vi "MAIN.vi"() -> ()   [LabVIEW 2020]
uses:
  GlobIndSw1.vi
panel:
  in  "Median Filter Rank":i32=25
  out "Oscilloscope Capture":waveform(dbl)[](graph)
  out "start time":timestamp
  out "Started":bool
  out "Elapsed time (minutes)":dbl
  out "error out":errorcluster
  in  "error in (no error)":errorcluster
  out "TEST#   |  Elapsed Time (minutes)":dbl[][](array[numeric])
  out "Inductive Switching :\nTotal Test Time (minutes)":dbl
  out "Cluster : Tf":cluster{"Tf (ns)":dbl, "DONE Tf":bool} {"Tf (ns)" format="%_12f"}
  out "Cluster : Tdoff":cluster{"Tdoff (ns)":dbl, "DONE Tdoff":bool} {"Tdoff (ns)" format="%_12f"}
  out "Cluster : Eoff":cluster{"Eoff (uj)":dbl, "DONE Eoff":bool} {"Eoff (uj)" format="%_12f"}
  out "Cluster : Dv/Dt ON":T1 {"Dv/Dt ON (V/us)" format="%_12f"}
  out "Cluster : Eon":cluster{"Eon (uj)":dbl, "DONE Eon":bool} {"Eon (uj)" format="%_12f"}
  out "Cluster : Di/Dt ON":T2 {"Di/Dt ON (A/us)" format="%_12f"}
  out "Cluster : Dv/DT OFF":T3 {"Dv/DT OFF (V/us)" format="%_12f"}
  out "Cluster : Di/Dt OFF":T4 {"Di/Dt OFF (A/us)" format="%_12f"}
  out "Cluster : Tr":cluster{"Tr (ns)":dbl, "DONE Tr":bool} {"Tr (ns)" format="%_12f"}
  out "Cluster : Tdon":cluster{"Tdon (ns)":dbl, "DONE Tdon":bool} {"Tdon (ns)" format="%_12f"}
  in  "Finish?":bool
  in  "Cluster : Setting":T5={"VGE (V)"=0.0, "VCE (V)"=0.0, "ICE (A)"=0.0, "TEKTRONIX"="", "PROJECT #"="", "TEMPERATURE (C)"=0.0, "RG (Ohm)"=0.0, "DUT #"=1, "REQUEST #"="", "TEST #"=1}
  out "CURRENT RESULT Array":dbl[](array[numeric])
  out "ALL RESULT Array":dbl[][](array[numeric])
  in  "START TEST":bool
  # "PRODUCED BY : AFIQAH HASBULLAH ( SBN CZ ENG : 2021)"
  # "AC MODULE : Inductive Switching"
  # "Column 2"
  # "Column 3"
  # "Column 4"
  # "Column 5"
  # "Column 6"
  # "Column 7"
  # "Column 8"
  # "Column 9"
  # "Column 10"
  # "Column 11"
  # "Column 12"
  # "Column 13"
  # "Column 14"
  # "Column 15"
  # "Column 16"
  # "Column 18"
  # "Column 19"
  # "Column 20"
  # "Column 21"
  # "Column 22"
  # "Column 23"
  # "Column 24"
  # "Column 25"
  # "Column 0"
  # "Column 1"
  # "----------------Already Calculated---------------------"
  # "Tdon\n(ns)"
  # "Tr\n(ns)"
  # "Tdoff\n(ns)"
  # "Tf\n(ns)"
  # "Eon\n(uj)"
  # "Eoff\n(uj)"
  # "di/dt (on)\nA/us"
  # "di/dt (off)\nA/us"
  # "dv/dt (on)\nV/us"
  # "dv/dt (off)\nV/us"
  # "NULL\n(Separator)"
  # "on\ndi (A)"
  # "on\ndt (ns)"
  # "off\ndi (A)"
  # "off\ndt (ns)"
  # "on\ndv (V)"
  # "on\ndt (ns)"
  # "off\ndv (V)"
  # "off\ndt (ns)"
  # "Vce"
  # "Ice"
  # "Vge"
  # "Rg"
  # "Temperature"
  # "DUT  #"
  # "TEST #"
  # "< Press 2 times >"
  # "Column 2"
  # "Column 3"
  # "Column 4"
  # "Column 5"
  # "Column 6"
  # "Column 7"
  # "Column 8"
  # "Column 9"
  # "Column 10"
  # "Column 11"
  # "Column 12"
  # "Column 13"
  # "Column 14"
  # "Column 15"
  # "Column 16"
  # "Column 18"
  # "Column 19"
  # "Column 20"
  # "Column 21"
  # "Column 22"
  # "Column 23"
  # "Column 24"
  # "Column 25"
  # "Column 0"
  # "Column 1"
  # "----------------Already Calculated---------------------"
  # "Tdon\n(ns)"
  # "Tr\n(ns)"
  # "Tdoff\n(ns)"
  # "Tf\n(ns)"
  # "Eon\n(uj)"
  # "Eoff\n(uj)"
  # "di/dt (on)\nA/us"
  # "di/dt (off)\nA/us"
  # "dv/dt (on)\nV/us"
  # "dv/dt (off)\nV/us"
  # "NULL\n(Separator)"
  # "on\ndi (A)"
  # "on\ndt (ns)"
  # "off\ndi (A)"
  # "off\ndt (ns)"
  # "on\ndv (V)"
  # "on\ndt (ns)"
  # "off\ndv (V)"
  # "off\ndt (ns)"
  # "TEST #"
  # "Vce"
  # "Ice"
  # "Vge"
  # "Rg"
  # "Temperature"
  # "DUT  #"
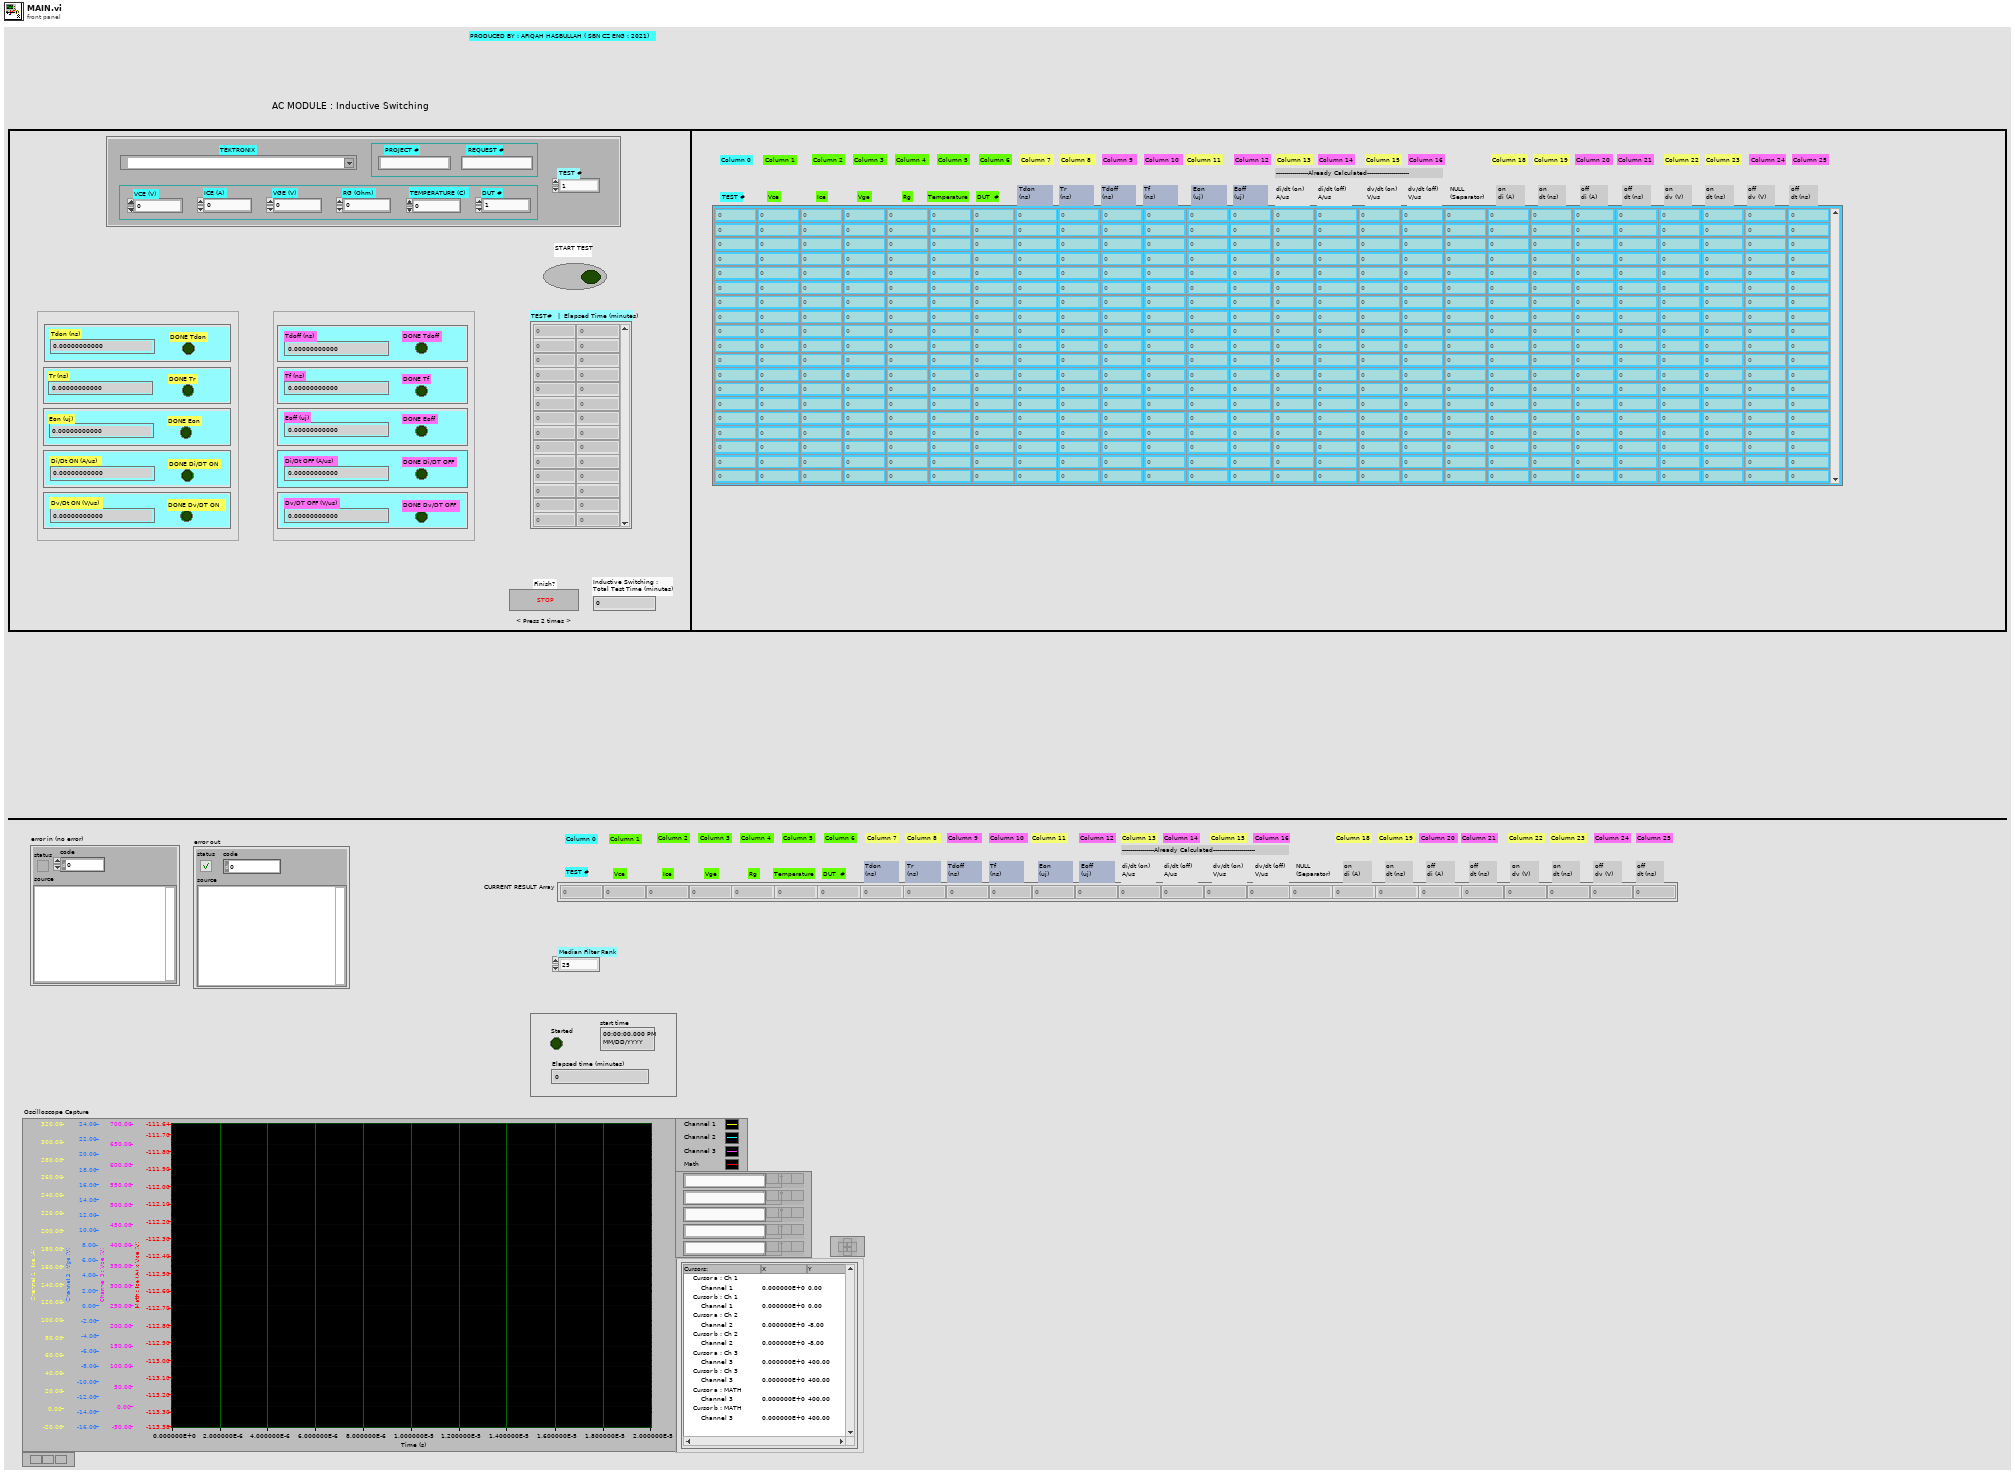
[diagram p1: front panel]
types:
  T1 = cluster{"Dv/Dt ON (V/us)":dbl, "DONE Dv/DT ON":bool}
  T2 = cluster{"Di/Dt ON (A/us)":dbl, "DONE Di/DT ON":bool}
  T3 = cluster{"Dv/DT OFF (V/us)":dbl, "DONE Dv/DT OFF":bool}
  T4 = cluster{"Di/Dt OFF (A/us)":dbl, "DONE Di/DT OFF":bool}
  T5 = cluster{"VGE (V)":dbl, "VCE (V)":dbl, "ICE (A)":dbl, "TEKTRONIX":refnum<visa-resource-name>, "PROJECT #":string, "TEMPERATURE (C)":dbl, "RG (Ohm)":dbl, "DUT #":i32, "REQUEST #":string, "TEST #":i32}
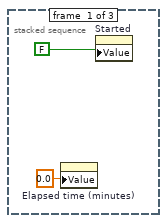
[diagram p2: hidden frame]
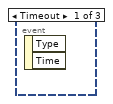
[diagram p4: hidden frame]
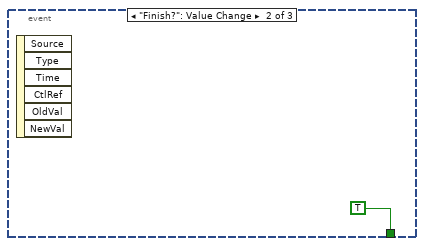
[diagram p5: hidden frame]
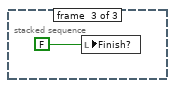
[diagram p7: hidden frame]
diagram:
  w23 = errorcluster {"status"=FALSE, "code"=0, "source"=""} ("error out")
  w4 = 0.0 ("Inductive Switching :\nTotal Test Time (minutes)")
  w5 = FALSE ("START TEST")
  w24 = cluster{"Tdon (ns)":dbl, "DONE Tdon":bool} {"Tdon (ns)"=0.0, "DONE Tdon"=FALSE} ("Cluster : Tdon")
  n1 = local read "Cluster : Setting"() -> (w19:T5)
  n2 = Bundle By Name(cluster=w19, "TEST #"=1, "DUT #"=1) -> (w20:T5)
  n3 = local write "Median Filter Rank"(25 ("Median Filter Rank")) -> ()
  n4 = local write "Cluster : Setting"(w20) -> ()
  n5 = flat-sequence {
    tunnel: [w26] -> w3
    tunnel: w3 -> [w27]
    tunnel: [w28] -> w22
    tunnel: w22 -> [w303]
    tunnel: [w301] -> w21
    tunnel: w21 -> [w328]
    frame #0 {
      # "IN"
      n6 = local read "error in (no error)"() -> (w26:errorcluster)
      n7 = Wait (ms)(milliseconds to wait=u32 100) -> ()  [unwired: 1 out]
    }
    frame #1 {
      # "Main Loop"
      n8 = while {
        shift-right: [w31] -> w28
        shift-left: w27 -> [w30]
        stop <- w33 stop-if-true
        n9 = local read "START TEST"() -> (w34:bool)
        n10 = case shown="True" w34 {
          tunnel: w30 -> [w35 w61]
          tunnel: [w35 w58] -> w31
          frame False {
          }
          frame True {
            # "Reset Start Button"
            # "Increment TEST# & DUT#"
            # "Update Data in All Result Array"
            # "OFF region Test"
            # "ON region Test"
            # "Header Information"
            # "Initialize"
            n11 = flat-sequence {
              tunnel: [w68] -> w62
              tunnel: w61 -> [w68]
              tunnel: [w93] -> w63
              tunnel: w62 -> [w93]
              tunnel: w63 -> [w148]
              tunnel: [w147] -> w57
              tunnel: [w126] -> w55
              tunnel: [w127] -> w54
              tunnel: [w128] -> w53
              tunnel: [w129] -> w52
              tunnel: [w136] -> w51
              tunnel: [w137] -> w50
              tunnel: [w135] -> w49
              tunnel: [w138] -> w48
              tunnel: [w139] -> w47
              tunnel: w57 -> [w199]
              tunnel: [w199] -> w56
              tunnel: w55 -> [w179]
              tunnel: w54 -> [w177]
              tunnel: w53 -> [w175]
              tunnel: w52 -> [w173]
              tunnel: w51 -> [w171]
              tunnel: w50 -> [w169]
              tunnel: w49 -> [w167]
              tunnel: w48 -> [w165]
              tunnel: w47 -> [w163]
              tunnel: w56 -> [w223]
              tunnel: [w222] -> w46
              tunnel: [w201] -> w44
              tunnel: [w202] -> w43
              tunnel: [w203] -> w42
              tunnel: [w204] -> w41
              tunnel: [w211] -> w40
              tunnel: [w212] -> w39
              tunnel: [w210] -> w38
              tunnel: [w213] -> w37
              tunnel: [w214] -> w36
              tunnel: w46 -> [w274]
              tunnel: [w274] -> w45
              tunnel: w44 -> [w254]
              tunnel: w43 -> [w252]
              tunnel: w42 -> [w250]
              tunnel: w41 -> [w248]
              tunnel: w40 -> [w246]
              tunnel: w39 -> [w244]
              tunnel: w38 -> [w242]
              tunnel: w37 -> [w240]
              tunnel: w36 -> [w238]
              tunnel: w45 -> [w277]
              tunnel: [w277] -> w59
              tunnel: [w283] -> w60
              tunnel: w59 -> [w283]
              tunnel: [w293] -> w58
              tunnel: w60 -> [w293]
              frame #0 {
                w69 = FALSE ("DONE Tdon")
                w70 = 0.0 ("Tdon (ns)")
                n12 = local read "Cluster : Di/Dt ON"() -> (w84:T2)
                n13 = local read "Cluster : Dv/Dt ON"() -> (w82:T1)
                n14 = local read "Cluster : Eon"() -> (w87:cluster{"Eon (uj)":dbl, "DONE Eon":bool})
                n15 = local read "Cluster : Tdon"() -> (w89:cluster{"Tdon (ns)":dbl, "DONE Tdon":bool})
                n16 = Bundle By Name(cluster=w84, "Di/Dt ON (A/us)"=w70, "DONE Di/DT ON"=w69) -> (w85:T2)
                n17 = local write "Oscilloscope Capture"(waveform(dbl)[] [] ("Oscilloscope Capture")) -> ()
                n18 = local read "Cluster : Tr"() -> (w90:cluster{"Tr (ns)":dbl, "DONE Tr":bool})
                n19 = Bundle By Name(cluster=w82, "Dv/Dt ON (V/us)"=w70, "DONE Dv/DT ON"=w69) -> (w83:T1)
                n20 = Bundle By Name(cluster=w87, "Eon (uj)"=w70, "DONE Eon"=w69) -> (w86:cluster{"Eon (uj)":dbl, "DONE Eon":bool})
                n21 = Bundle By Name(cluster=w89, "Tdon (ns)"=w70, "DONE Tdon"=w69) -> (w88:cluster{"Tdon (ns)":dbl, "DONE Tdon":bool})
                n22 = Bundle By Name(cluster=w90, "Tr (ns)"=w70, "DONE Tr"=w69) -> (w91:cluster{"Tr (ns)":dbl, "DONE Tr":bool})
                n23 = local write "Cluster : Di/Dt ON"(w85) -> ()
                n24 = local write "Cluster : Dv/Dt ON"(w83) -> ()
                n25 = local write "Cluster : Eon"(w86) -> ()
                n26 = local write "Cluster : Tdon"(w88) -> ()
                n27 = local write "Cluster : Tr"(w91) -> ()
                n28 = Initialize Array(0.0 ("element"), 26 ("dimension size")) -> (w65:dbl[])
                n29 = local write "CURRENT RESULT Array"(w65) -> ()
                n30 = local read "Cluster : Di/Dt OFF"() -> (w77:T4)
                n31 = local read "Cluster : Tdoff"() -> (w74:cluster{"Tdoff (ns)":dbl, "DONE Tdoff":bool})
                n32 = local read "Cluster : Eoff"() -> (w76:cluster{"Eoff (uj)":dbl, "DONE Eoff":bool})
                n33 = local read "Cluster : Tf"() -> (w71:cluster{"Tf (ns)":dbl, "DONE Tf":bool})
                n34 = local read "Cluster : Dv/DT OFF"() -> (w80:T3)
                n35 = Bundle By Name(cluster=w77, "Di/Dt OFF (A/us)"=w70, "DONE Di/DT OFF"=w69) -> (w78:T4)
                n36 = Bundle By Name(cluster=w74, "Tdoff (ns)"=w70, "DONE Tdoff"=w69) -> (w73:cluster{"Tdoff (ns)":dbl, "DONE Tdoff":bool})
                n37 = Bundle By Name(cluster=w76, "Eoff (uj)"=w70, "DONE Eoff"=w69) -> (w75:cluster{"Eoff (uj)":dbl, "DONE Eoff":bool})
                n38 = Bundle By Name(cluster=w71, "Tf (ns)"=w70, "DONE Tf"=w69) -> (w72:cluster{"Tf (ns)":dbl, "DONE Tf":bool})
                n39 = Bundle By Name(cluster=w80, "Dv/DT OFF (V/us)"=w70, "DONE Dv/DT OFF"=w69) -> (w79:T3)
                n40 = local write "Cluster : Tdoff"(w73) -> ()
                n41 = local write "Cluster : Di/Dt OFF"(w78) -> ()
                n42 = local write "Cluster : Eoff"(w75) -> ()
                n43 = local write "Cluster : Tf"(w72) -> ()
                n44 = local write "Cluster : Dv/DT OFF"(w79) -> ()
                n45 = Wait (ms)(milliseconds to wait=u32 400) -> ()  [unwired: 1 out]
              }
              frame #1 {
                # "Column 6 = DUT#"
                # "Column 5 = Temperature"
                # "Column 4 = RG"
                # "Column 3 = VGE"
                # "Column 2 = ICE"
                # "Column 1 = VCE"
                # "Column 0 = TEST#"
                n46 = local read "Cluster : Setting"() -> (w123:T5)
                n47 = Wait (ms)(milliseconds to wait=u32 400) -> ()  [unwired: 1 out]
                n48 = Unbundle By Name(w123) -> ("TEST #"=w119:i32, "ICE (A)"=w111:dbl, "VGE (V)"=w107:dbl, "VCE (V)"=w115:dbl, "RG (Ohm)"=w103:dbl, "TEMPERATURE (C)"=w99:dbl, "DUT #"=w95:i32)
                n49 = local read "CURRENT RESULT Array"() -> (w122:dbl[])
                n50 = local read "CURRENT RESULT Array"() -> (w116:dbl[])
                n51 = local read "CURRENT RESULT Array"() -> (w114:dbl[])
                n52 = local read "Median Filter Rank"() -> (w92:i32)
                n53 = local read "CURRENT RESULT Array"() -> (w108:dbl[])
                n54 = local read "CURRENT RESULT Array"() -> (w106:dbl[])
                n55 = local read "CURRENT RESULT Array"() -> (w100:dbl[])
                n56 = local read "CURRENT RESULT Array"() -> (w98:dbl[])
                n57 = Replace Array Subset(array=w122, new element=w119, index=0) -> (w121:dbl[])
                n58 = Replace Array Subset(array=w116, new element=w115, index=1) -> (w117:dbl[])
                n59 = Replace Array Subset(array=w114, new element=w111, index=2) -> (w113:dbl[])
                n60 = global write "GlobIndSw1.vi" "Median Filter Rank"(w92) -> ()
                n61 = Replace Array Subset(array=w108, new element=w107, index=3) -> (w109:dbl[])
                n62 = Replace Array Subset(array=w106, new element=w103, index=4) -> (w105:dbl[])
                n63 = Replace Array Subset(array=w100, new element=w99, index=5) -> (w101:dbl[])
                n64 = Replace Array Subset(array=w98, new element=w95, index=6) -> (w97:dbl[])
                n65 = local write "CURRENT RESULT Array"(w121) -> ()
                n66 = local write "CURRENT RESULT Array"(w117) -> ()
                n67 = local write "CURRENT RESULT Array"(w113) -> ()
                n68 = local write "CURRENT RESULT Array"(w109) -> ()
                n69 = local write "CURRENT RESULT Array"(w105) -> ()
                n70 = local write "CURRENT RESULT Array"(w101) -> ()
                n71 = local write "CURRENT RESULT Array"(w97) -> ()
              }
              frame #2 {
                n72 = local read "Cluster : Setting"() -> (w161:T5)
                n73 = Unbundle By Name(w161) -> ("TEKTRONIX"=w146:refnum<visa-resource-name>, "PROJECT #"=w145:string, "REQUEST #"=w144:string, "TEST #"=w150:i32, "ICE (A)"=w142:dbl, "VGE (V)"=w141:dbl, "VCE (V)"=w140:dbl)
                n74 = Format Value(format string="%d", value (0)=w150) -> (output string=w143:string)  [unwired: 1 in]
                n75 = call "f_ON_Region.vi"("VISA Resource Name"=w146, "Project #"=w145, "Request #"=w144, "TEST #"=w143, "ICE"=w142, "VGE"=w141, "VCE"=w140, "error in (no error)"=w148) -> ("Tdon (ns)"=w139:dbl, "Di (A)"=w129:dbl, "Tr (ns)"=w138:dbl, "Dt (ns)"=w128:dbl, "Di/Dt (A/us)"=w137:dbl, "Dv/Dt (V/us)"=w136:dbl, "Eon (uj)"=w135:dbl, "Dv (V)"=w127:dbl, "Dt (ns) 2"=w126:dbl, "DONE Tdon"=w134:bool, "DONE Tr"=w133:bool, "DONE Di/Dt ON"=w132:bool, "DONE Dv/Dt ON"=w131:bool, "DONE Eon"=w130:bool, "Oscilloscope Capture"=w124:waveform(dbl)[], "error out"=w147:errorcluster)  [unwired: 4 in]
                n76 = local write "Oscilloscope Capture"(w124) -> ()
                n77 = local read "Cluster : Dv/Dt ON"() -> (w160:T1)
                n78 = local read "Cluster : Di/Dt ON"() -> (w158:T2)
                n79 = Bundle By Name(cluster=w160, "Dv/Dt ON (V/us)"=w136, "DONE Dv/DT ON"=w131) -> (w159:T1)
                n80 = Bundle By Name(cluster=w158, "Di/Dt ON (A/us)"=w137, "DONE Di/DT ON"=w132) -> (w157:T2)
                n81 = local read "Cluster : Eon"() -> (w155:cluster{"Eon (uj)":dbl, "DONE Eon":bool})
                n82 = local read "Cluster : Tr"() -> (w152:cluster{"Tr (ns)":dbl, "DONE Tr":bool})
                n83 = local read "Cluster : Tdon"() -> (w153:cluster{"Tdon (ns)":dbl, "DONE Tdon":bool})
                n84 = Bundle By Name(cluster=w155, "Eon (uj)"=w135, "DONE Eon"=w130) -> (w156:cluster{"Eon (uj)":dbl, "DONE Eon":bool})
                n85 = Bundle By Name(cluster=w152, "Tr (ns)"=w138, "DONE Tr"=w133) -> (w151:cluster{"Tr (ns)":dbl, "DONE Tr":bool})
                n86 = Bundle By Name(cluster=w153, "Tdon (ns)"=w139, "DONE Tdon"=w134) -> (w154:cluster{"Tdon (ns)":dbl, "DONE Tdon":bool})
                n87 = local write "Cluster : Dv/Dt ON"(w159) -> ()
                n88 = local write "Cluster : Di/Dt ON"(w157) -> ()
                n89 = local write "Cluster : Eon"(w156) -> ()
                n90 = local write "Cluster : Tr"(w151) -> ()
                n91 = local write "Cluster : Tdon"(w154) -> ()
                n92 = Wait (ms)(milliseconds to wait=u32 300) -> ()  [unwired: 1 out]
              }
              frame #3 {
                # "Column 23 = Dt2"
                # "Column 22 = Dv"
                # "Column 19 = Dt"
                # "Column 18 = Di"
                # "Column 15 = DvDtON"
                # "Column 13 = DiDtON"
                # "Column 11 = Eon"
                # "Column 8 = Tr"
                # "Column 7 = Tdon"
                n93 = Wait (ms)(milliseconds to wait=u32 2000) -> ()  [unwired: 1 out]
                n94 = local read "CURRENT RESULT Array"() -> (w181:dbl[])
                n95 = local read "CURRENT RESULT Array"() -> (w184:dbl[])
                n96 = local read "CURRENT RESULT Array"() -> (w188:dbl[])
                n97 = local read "CURRENT RESULT Array"() -> (w185:dbl[])
                n98 = local read "CURRENT RESULT Array"() -> (w189:dbl[])
                n99 = local read "CURRENT RESULT Array"() -> (w197:dbl[])
                n100 = local read "CURRENT RESULT Array"() -> (w193:dbl[])
                n101 = local read "CURRENT RESULT Array"() -> (w196:dbl[])
                n102 = local read "CURRENT RESULT Array"() -> (w192:dbl[])
                n103 = Replace Array Subset(array=w181, new element=w163, index=7) -> (w182:dbl[])
                n104 = Replace Array Subset(array=w184, new element=w165, index=8) -> (w183:dbl[])
                n105 = Replace Array Subset(array=w188, new element=w169, index=13) -> (w187:dbl[])
                n106 = Replace Array Subset(array=w185, new element=w167, index=11) -> (w186:dbl[])
                n107 = Replace Array Subset(array=w189, new element=w171, index=15) -> (w190:dbl[])
                n108 = Replace Array Subset(array=w197, new element=w173, index=18) -> (w198:dbl[])
                n109 = Replace Array Subset(array=w193, new element=w177, index=22) -> (w194:dbl[])
                n110 = Replace Array Subset(array=w196, new element=w175, index=19) -> (w195:dbl[])
                n111 = Replace Array Subset(array=w192, new element=w179, index=23) -> (w191:dbl[])
                n112 = local write "CURRENT RESULT Array"(w182) -> ()
                n113 = local write "CURRENT RESULT Array"(w183) -> ()
                n114 = local write "CURRENT RESULT Array"(w187) -> ()
                n115 = local write "CURRENT RESULT Array"(w186) -> ()
                n116 = local write "CURRENT RESULT Array"(w190) -> ()
                n117 = local write "CURRENT RESULT Array"(w198) -> ()
                n118 = local write "CURRENT RESULT Array"(w194) -> ()
                n119 = local write "CURRENT RESULT Array"(w195) -> ()
                n120 = local write "CURRENT RESULT Array"(w191) -> ()
              }
              frame #4 {
                n121 = local read "Cluster : Setting"() -> (w225:T5)
                n122 = Unbundle By Name(w225) -> ("TEKTRONIX"=w221:refnum<visa-resource-name>, "PROJECT #"=w220:string, "REQUEST #"=w219:string, "TEST #"=w236:i32, "ICE (A)"=w217:dbl, "VGE (V)"=w216:dbl, "VCE (V)"=w215:dbl)
                n123 = Format Value(format string="%d", value (0)=w236) -> (output string=w218:string)  [unwired: 1 in]
                n124 = call "f_OFF_Region.vi"("VISA Resource Name"=w221, "Project #"=w220, "Request #"=w219, "TEST #"=w218, "ICE"=w217, "VGE"=w216, "VCE"=w215, "error in (no error)"=w223) -> ("Tdoff (ns)"=w214:dbl, "Di (A)"=w204:dbl, "Tf (ns)"=w213:dbl, "Dt (ns)"=w203:dbl, "Di/Dt (A/us)"=w212:dbl, "Dv/Dt (V/us)"=w211:dbl, "Eoff (uj)"=w210:dbl, "Dv (V)"=w202:dbl, "Dt (ns) 2"=w201:dbl, "DONE Tdoff"=w209:bool, "DONE Tf"=w208:bool, "DONE Di/Dt OFF"=w207:bool, "DONE Dv/Dt OFF"=w206:bool, "DONE Eoff"=w205:bool, "error out"=w222:errorcluster)  [unwired: 5 in]
                n125 = local read "Cluster : Dv/DT OFF"() -> (w226:T3)
                n126 = local read "Cluster : Di/Dt OFF"() -> (w228:T4)
                n127 = Bundle By Name(cluster=w226, "Dv/DT OFF (V/us)"=w211, "DONE Dv/DT OFF"=w206) -> (w227:T3)
                n128 = Bundle By Name(cluster=w228, "Di/Dt OFF (A/us)"=w212, "DONE Di/DT OFF"=w207) -> (w229:T4)
                n129 = local read "Cluster : Eoff"() -> (w231:cluster{"Eoff (uj)":dbl, "DONE Eoff":bool})
                n130 = local read "Cluster : Tf"() -> (w234:cluster{"Tf (ns)":dbl, "DONE Tf":bool})
                n131 = local read "Cluster : Tdoff"() -> (w233:cluster{"Tdoff (ns)":dbl, "DONE Tdoff":bool})
                n132 = Bundle By Name(cluster=w231, "Eoff (uj)"=w210, "DONE Eoff"=w205) -> (w230:cluster{"Eoff (uj)":dbl, "DONE Eoff":bool})
                n133 = Bundle By Name(cluster=w234, "Tf (ns)"=w213, "DONE Tf"=w208) -> (w235:cluster{"Tf (ns)":dbl, "DONE Tf":bool})
                n134 = Bundle By Name(cluster=w233, "Tdoff (ns)"=w214, "DONE Tdoff"=w209) -> (w232:cluster{"Tdoff (ns)":dbl, "DONE Tdoff":bool})
                n135 = local write "Cluster : Dv/DT OFF"(w227) -> ()
                n136 = local write "Cluster : Di/Dt OFF"(w229) -> ()
                n137 = local write "Cluster : Eoff"(w230) -> ()
                n138 = local write "Cluster : Tf"(w235) -> ()
                n139 = local write "Cluster : Tdoff"(w232) -> ()
                n140 = Wait (ms)(milliseconds to wait=u32 300) -> ()  [unwired: 1 out]
              }
              frame #5 {
                # "Column 25 = Dt2"
                # "Column 24 = Dv"
                # "Column 21 = Dt"
                # "Column 20 = Di"
                # "Column 16 = DvDtOFF"
                # "Column 14 = DiDtOFF"
                # "Column 12 = Eoff"
                # "Column 10 = Tf"
                # "Column 9 = Tdoff"
                n141 = Wait (ms)(milliseconds to wait=u32 2000) -> ()  [unwired: 1 out]
                n142 = local read "CURRENT RESULT Array"() -> (w273:dbl[])
                n143 = local read "CURRENT RESULT Array"() -> (w270:dbl[])
                n144 = local read "CURRENT RESULT Array"() -> (w266:dbl[])
                n145 = local read "CURRENT RESULT Array"() -> (w269:dbl[])
                n146 = local read "CURRENT RESULT Array"() -> (w265:dbl[])
                n147 = local read "CURRENT RESULT Array"() -> (w257:dbl[])
                n148 = local read "CURRENT RESULT Array"() -> (w261:dbl[])
                n149 = local read "CURRENT RESULT Array"() -> (w258:dbl[])
                n150 = local read "CURRENT RESULT Array"() -> (w262:dbl[])
                n151 = Replace Array Subset(array=w273, new element=w238, index=9) -> (w272:dbl[])
                n152 = Replace Array Subset(array=w270, new element=w240, index=10) -> (w271:dbl[])
                n153 = Replace Array Subset(array=w266, new element=w244, index=14) -> (w267:dbl[])
                n154 = Replace Array Subset(array=w269, new element=w242, index=12) -> (w268:dbl[])
                n155 = Replace Array Subset(array=w265, new element=w246, index=16) -> (w264:dbl[])
                n156 = Replace Array Subset(array=w257, new element=w248, index=20) -> (w256:dbl[])
                n157 = Replace Array Subset(array=w261, new element=w252, index=24) -> (w260:dbl[])
                n158 = Replace Array Subset(array=w258, new element=w250, index=21) -> (w259:dbl[])
                n159 = Replace Array Subset(array=w262, new element=w254, index=25) -> (w263:dbl[])
                n160 = local write "CURRENT RESULT Array"(w272) -> ()
                n161 = local write "CURRENT RESULT Array"(w271) -> ()
                n162 = local write "CURRENT RESULT Array"(w267) -> ()
                n163 = local write "CURRENT RESULT Array"(w268) -> ()
                n164 = local write "CURRENT RESULT Array"(w264) -> ()
                n165 = local write "CURRENT RESULT Array"(w256) -> ()
                n166 = local write "CURRENT RESULT Array"(w260) -> ()
                n167 = local write "CURRENT RESULT Array"(w259) -> ()
                n168 = local write "CURRENT RESULT Array"(w263) -> ()
              }
              frame #6 {
                n169 = local read "Cluster : Setting"() -> (w282:T5)
                n170 = Unbundle By Name(w282) -> ("TEST #"=w276:i32)
                n171 = local read "CURRENT RESULT Array"() -> (w281:dbl[])
                n172 = local read "ALL RESULT Array"() -> (w280:dbl[][])
                n173 = Decrement(x=w276) -> (x-1=w275:i32)
                n174 = Replace Array Subset(array=w280, new element=w281, index (row)=w275) -> (w279:dbl[][])  [unwired: 1 in]
                n175 = local write "ALL RESULT Array"(w279) -> ()
                n176 = Wait (ms)(milliseconds to wait=u32 300) -> ()  [unwired: 1 out]
              }
              frame #7 {
                n177 = local read "Cluster : Setting"() -> (w291:T5)
                n178 = Unbundle By Name(w291) -> ("TEST #"=w290:i32, "DUT #"=w289:i32)
                n179 = Increment(x=w290) -> (x+1=w285:i32)
                n180 = Increment(x=w289) -> (x+1=w284:i32)
                n181 = local read "Cluster : Setting"() -> (w287:T5)
                n182 = Bundle By Name(cluster=w287, "TEST #"=w285, "DUT #"=w284) -> (w286:T5)
                n183 = local write "Cluster : Setting"(w286) -> ()
                n184 = Wait (ms)(milliseconds to wait=u32 200) -> ()  [unwired: 1 out]
              }
              frame #8 {
                n185 = local write "START TEST"(FALSE ("START TEST")) -> ()
                n186 = local write "Started"(FALSE ("START TEST")) -> ()
                n187 = Wait (ms)(milliseconds to wait=u32 1000) -> ()  [unwired: 1 out]
              }
            }
          }
        }
        n188 = Wait (ms)(milliseconds to wait=u32 100) -> ()  [unwired: 1 out]
        n189 = local read "Finish?"() -> (w33:bool)
      }
      n190 = Wait (ms)(milliseconds to wait=u32 100) -> ()  [unwired: 1 out]
    }
    frame #2 {
      # "Minutes"
      # "Export to Excel"
      n191 = local read "TEST#   |  Elapsed Time (minutes)"() -> (w308:dbl[][])
      n192 = local read "Cluster : Setting"() -> (w315:T5)
      n193 = Unbundle By Name(w315) -> ("TEST #"=w297:i32)
      n194 = Index Array(array=w308, index (col)=1 ("disabled index (col)")) -> (element=w306:dbl[])  [unwired: 1 in]
      n195 = Decrement(x=w297) -> (x-1=w296:i32)
      n196 = local read "ALL RESULT Array"() -> (w310:dbl[][])
      n197 = local read "Cluster : Setting"() -> (w319:T5)
      n198 = Split 1D Array(array=w306, index=w296) -> (first subarray=w305:dbl[])  [unwired: 1 out]
      n199 = Decrement(x=w297) -> (x-1=w311:i32)
      n200 = for {
        tunnel: w305 -> [w323] mode=indexing
        shift-right: [w322] -> w304
        shift-left: 0.0 -> [w321]
        shift-right: [w320] -> w300
        shift-left: w303 -> [w320]
        n201 = Add(x=w323, y=w321) -> (x+y=w322:dbl)
        n202 = local write "Inductive Switching :\nTotal Test Time (minutes)"(w322) -> ()
      }
      n203 = Unbundle By Name(w319) -> ("PROJECT #"=w318:string, "REQUEST #"=w317:string)
      n204 = Array Subset(array=w310, index (row)=0 ("index"), length (row)=w311, index (col)=0 ("index"), length (col)=26 ("length")) -> (w309:dbl[][])
      n205 = call "O_Data_to_Excel.vi"("error in (no error)"=w303, "ALL RESULT Array"=w309, "REQUEST #"=w317, "PROJECT #"=w318) -> ("error out"=w299:errorcluster)  [unwired: 7 in]
      n206 = Wait (ms)(milliseconds to wait=u32 100) -> ()  [unwired: 1 out]
      n207 = local write "Inductive Switching :\nTotal Test Time (minutes)"(w304) -> ()
      n208 = Merge Errors(w299, w300) -> (w298:errorcluster)
      n209 = while {
        shift-right: [w324] -> w301
        shift-left: w298 -> [w325]
        stop <- w326 stop-if-true
        n210 = call "Display Message to User"("error in (no error)"=w325) -> ("error out"=w324:errorcluster, "OK"=w326:bool)  [unwired: 9 in]
        n211 = Wait (ms)(milliseconds to wait=u32 100) -> ()  [unwired: 1 out]
      }
    }
    frame #3 {
      # "OUT"
      n212 = local write "error out"(w328) -> ()
      n213 = Wait (ms)(milliseconds to wait=u32 100) -> ()  [unwired: 1 out]
    }
  }
  n214 = Initialize Array(0.0 ("element"), 26 ("dimension size")) -> (→"CURRENT RESULT Array":dbl[])
  n215 = Initialize Array(0.0 ("element"), 100 ("dimension size"), 2 ("dimension size")) -> (→"TEST#   |  Elapsed Time (minutes)":dbl[][])
  n216 = Initialize Array(0.0 ("element"), 100 ("dimension size"), 26 ("dimension size")) -> (→"ALL RESULT Array":dbl[][])
  n217 = local write "Started"(w5) -> ()
  n218 = local write "START TEST"(w5) -> ()
  n219 = local write "Finish?"(w5) -> ()
  n220 = local write "error out"(w23) -> ()
  n221 = local write "error in (no error)"(w23) -> ()
  n222 = while {
    stop <- w331 stop-if-true
    # "COPY from NI Forum :)"
    n223 = stacked-sequence {
      tunnel: [_ w334 _] -> w331
      frame #0 {
        n224 = property on="Elapsed time (minutes)" class="DigNum (strict)"("Value"=0.0 ("Elapsed time (seconds)")) -> ()  [unwired: 2 in, 2 out]
        n225 = property on="Started" class="Bool (strict)"("Value"=FALSE ("Started")) -> ()  [unwired: 2 in, 2 out]
      }
      frame #1 {
        n226 = while {
          tunnel: [w335] -> w334
          stop <- w335 stop-if-true
          n227 = local read "Started"() -> (w336:bool)
          n228 = case shown="True" w336 {
            frame False {
              # "do nothing"
            }
            frame True {
              n229 = local read "start time"() -> (w348:timestamp)
              n230 = local read "Cluster : Setting"() -> (w344:T5)
              n231 = Get Date/Time In Seconds() -> (seconds since 1Jan1904=w347:timestamp)
              n232 = Subtract(x=w347, y=w348) -> (x-y=w346:dbl)
              n233 = Divide(x=w346, y=60.0) -> (x/y=w338:dbl)
              n234 = Unbundle By Name(w344) -> ("TEST #"=w340:i32)
              n235 = local write "Elapsed time (minutes)"(w338) -> ()
              n236 = Build Array(w340, w338) -> (w341:dbl[])
              n237 = local read "TEST#   |  Elapsed Time (minutes)"() -> (w343:dbl[][])
              n238 = Decrement(x=w340) -> (x-1=w339:i32)
              n239 = Replace Array Subset(array=w343, new element=w341, index (row)=w339) -> (w342:dbl[][])  [unwired: 1 in]
              n240 = local write "TEST#   |  Elapsed Time (minutes)"(w342) -> ()
            }
          }
          n241 = local read "Finish?"() -> (w335:bool)
          n242 = Wait (ms)(milliseconds to wait=u32 10) -> ()  [unwired: 1 out]
        }
        n243 = while {
          stop <- w349 stop-if-true
          n244 = event shown="[2] \"START TEST\": Value Change" {
            selector: _ -> [_ _ _]
            dyn-events: _ -> [_ _ _]
            timeout: _ -> [_ _ _]
            tunnel: [_ TRUE FALSE] -> w349
            event Timeout {
              n245 = event-data() -> ()  [unwired: 1 in, 2 out]
            }
            event "Finish?": Value Change {
              n246 = event-data() -> ()  [unwired: 1 in, 6 out]
            }
            event "START TEST": Value Change {
              n247 = event-data() -> ()  [unwired: 1 in, 6 out]
              n248 = local read "Started"() -> (w353:bool)
              n249 = Not(x=w353) -> (.not. x?=w351:bool)
              n250 = case shown="True" w351 {
                frame False {
                }
                frame True {
                  n251 = Get Date/Time In Seconds() -> (seconds since 1Jan1904=→"start time":timestamp)
                }
              }
              n252 = local write "Started"(w351) -> ()
            }
          }
        }
      }
      frame #2 {
        n253 = local write "Finish?"(FALSE ("stop")) -> ()
      }
    }
    n254 = Wait (ms)(milliseconds to wait=u32 100) -> ()  [unwired: 1 out]
  }
  "Cluster : Tdon" <- w24
  "Cluster : Tr" <- w24
  "Cluster : Di/Dt OFF" <- w24
  "Cluster : Dv/DT OFF" <- w24
  "Cluster : Di/Dt ON" <- w24
  "Cluster : Eon" <- w24
  "Cluster : Dv/Dt ON" <- w24
  "Cluster : Eoff" <- w24
  "Cluster : Tdoff" <- w24
  "Cluster : Tf" <- w24
  "Inductive Switching :\nTotal Test Time (minutes)" <- w4
  "Elapsed time (minutes)" <- w4
  "Oscilloscope Capture" <- waveform(dbl)[] [] ("Oscilloscope Capture")
